vi "PS Control Write v0.80.vi"(4 "FRTZ":bool, 5 "Pause":bool, 6 "stop":bool, 7 "Ramp":bool=TRUE, 8 "error in (no error)":errorcluster, 9 "Slew Rate":dbl(slide)=10.0 scale=0.2..600.0 scale format="%.1f", 10 "Setpoint":dbl format="%.2f", 11 "Units":bool caption="tesla            kAmps") -> (0 "error out":errorcluster, 3 "Time(ms)":u32)   [LabVIEW 2024]
panel:
  # "(To Zero Goes\nTo 100 A)"
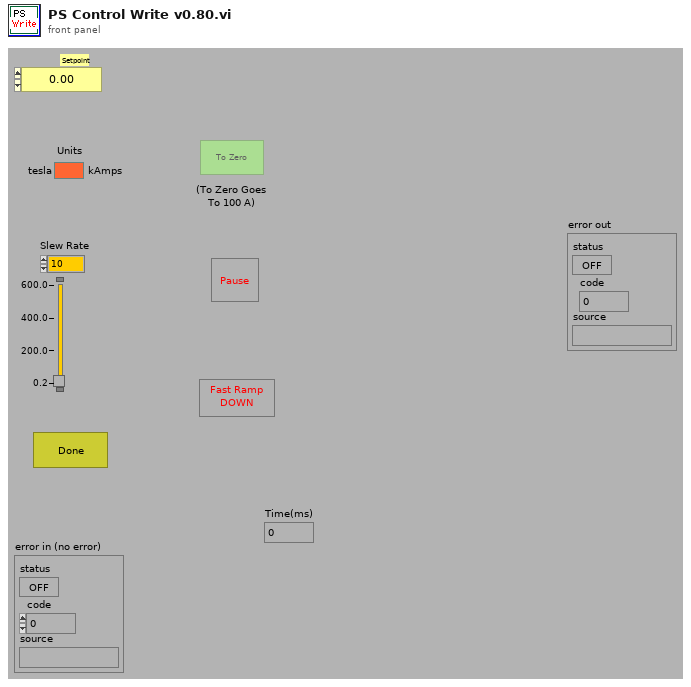
[diagram p1: front panel]
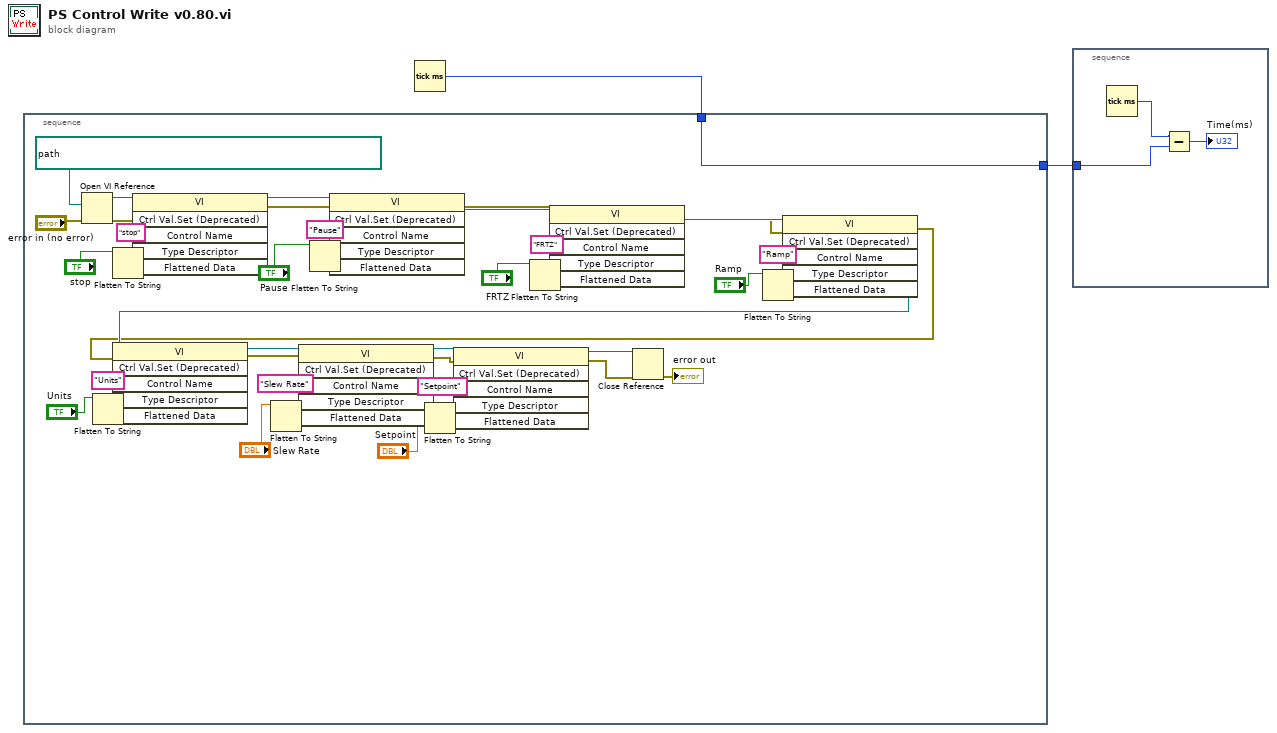
[diagram p0: block diagram]
diagram:
  n1 = Tick Count (ms)() -> (millisecond timer value=w2:u32)
  n2 = stacked-sequence {
    tunnel: [w15] -> w1
    tunnel: w2 -> [w15]
    frame #0 {
      n3 = Open VI Reference(vi path=path "/Optics2Mac/xwei Work/NML Data Acq/Serial Instruments/PS ƒ\n/PS Control", error in (no error)="error in (no error)") -> (vi reference=w36:refnum<vi>, error out=w3:errorcluster)  [unwired: 4 in]
      n4 = Flatten To String(anything="Units") -> (data string=w49:string, type string=w48:i16[])  [unwired: 3 in, 1 out]
      n5 = Flatten To String(anything="stop") -> (data string=w33:string, type string=w34:i16[])  [unwired: 3 in, 1 out]
      n6 = invoke class="VI" method="Ctrl Val.Set (Deprecated)"(reference=w36, error in=w3, "Control Name"="stop", "Type Descriptor"=w34, "Flattened Data"=w33) -> (reference out=w19:refnum<vi>, error out=w11:errorcluster)  [unwired: 1 in, 4 out]
      n7 = Flatten To String(anything="Slew Rate") -> (data string=w40:string, type string=w41:i16[])  [unwired: 3 in, 1 out]
      n8 = Flatten To String(anything="Pause") -> (data string=w21:string, type string=w22:i16[])  [unwired: 3 in, 1 out]
      n9 = invoke class="VI" method="Ctrl Val.Set (Deprecated)"(reference=w19, error in=w11, "Control Name"="Pause", "Type Descriptor"=w22, "Flattened Data"=w21) -> (reference out=w18:refnum<vi>, error out=w10:errorcluster)  [unwired: 1 in, 4 out]
      n10 = Flatten To String(anything="Setpoint") -> (data string=w43:string, type string=w44:i16[])  [unwired: 3 in, 1 out]
      n11 = Flatten To String(anything="FRTZ") -> (data string=w30:string, type string=w31:i16[])  [unwired: 3 in, 1 out]
      n12 = invoke class="VI" method="Ctrl Val.Set (Deprecated)"(reference=w18, error in=w10, "Control Name"="FRTZ", "Type Descriptor"=w31, "Flattened Data"=w30) -> (reference out=w17:refnum<vi>, error out=w9:errorcluster)  [unwired: 1 in, 4 out]
      n13 = Flatten To String(anything="Ramp") -> (data string=w27:string, type string=w28:i16[])  [unwired: 3 in, 1 out]
      n14 = invoke class="VI" method="Ctrl Val.Set (Deprecated)"(reference=w17, error in=w9, "Control Name"="Ramp", "Type Descriptor"=w28, "Flattened Data"=w27) -> (reference out=w16:refnum<vi>, error out=w8:errorcluster)  [unwired: 1 in, 4 out]
      n15 = invoke class="VI" method="Ctrl Val.Set (Deprecated)"(reference=w16, error in=w8, "Control Name"="Units", "Type Descriptor"=w48, "Flattened Data"=w49) -> (reference out=w37:refnum<vi>, error out=w7:errorcluster)  [unwired: 1 in, 4 out]
      n16 = invoke class="VI" method="Ctrl Val.Set (Deprecated)"(reference=w37, error in=w7, "Control Name"="Slew Rate", "Type Descriptor"=w41, "Flattened Data"=w40) -> (reference out=w38:refnum<vi>, error out=w6:errorcluster)  [unwired: 1 in, 4 out]
      n17 = invoke class="VI" method="Ctrl Val.Set (Deprecated)"(reference=w38, error in=w6, "Control Name"="Setpoint", "Type Descriptor"=w44, "Flattened Data"=w43) -> (reference out=w13:refnum<vi>, error out=w5:errorcluster)  [unwired: 1 in, 4 out]
      n18 = Close Reference(reference=w13, error in (no error)=w5) -> (error out=→"error out":errorcluster)
    }
  }
  n19 = stacked-sequence {
    tunnel: w1 -> [w52]
    frame #0 {
      n20 = Tick Count (ms)() -> (millisecond timer value=w53:u32)
      n21 = Subtract(x=w53, y=w52) -> (x-y=→"Time(ms)":u32)
    }
  }
